vi "test_ServiceLocationPool_GetInvalidServiceTwice_DoesNotCacheInvalidData.vi"(8 "error in (no error)":errorcluster) -> (0 "error out":errorcluster, 2 "result":string, 3 "pass":bool)   [LabVIEW 2020, in "MeasurementServerTests.lvlib"]
uses:
  MeasurementServerTests.lvlib
  Runtime/MeasurementLink Discovery/MeasurementLink Discovery.lvlib
  Runtime/MeasurementLink Discovery Client/RPC Messages/ni_measurementlink_discovery_v1_ResolveServiceRequest.ctl
  Runtime/MeasurementLink Discovery Client/MeasurementLink Discovery Client.lvlib
  Runtime/MeasurementLink Discovery/Service Location FGV Action.ctl
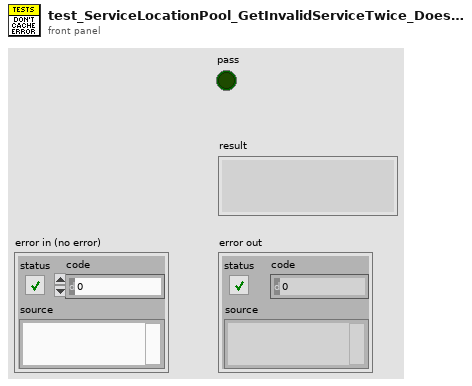
[diagram p1: front panel]
types:
  T1 = typedef "MeasurementLink Discovery Client.lvlib/ni_measurementlink_discovery_v1_ResolveServiceRequest.ctl" = cluster{"provided_interface":string, "service_class":string}
  T2 = typedef "MeasurementLink Discovery.lvlib/Service Location FGV Action.ctl" = enum16{"Get Service Location", "Reresolve Service Location"}
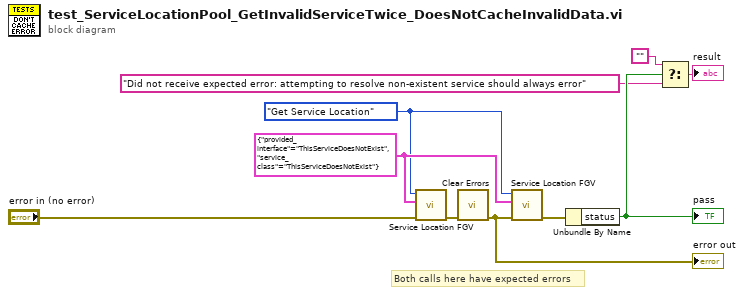
[diagram p0: block diagram]
diagram:
  w9 = T1 {"provided_interface"="ThisServiceDoesNotExist", "service_class"="ThisServiceDoesNotExist"} ("Resolve Service Request")
  w8 = Service_Location_FGV_Action."Get Service Location" ("Action")
  # "Both calls here have expected errors"
  n1 = call "Service Location FGV.vi"("error in"="error in (no error)", "resolve service request"=w9, "action"=w8) -> ("error out"=w6:errorcluster)  [unwired: 6 in, 2 out]
  n2 = call <vilib>:"Clear Errors.vi"("error in (no error)"=w6) -> ("error out"=w1:errorcluster)  [unwired: 5 in, 1 out]
  "error out" <- w1
  n3 = call "Service Location FGV.vi"("error in"=w1, "resolve service request"=w9, "action"=w8) -> ("error out"=w5:errorcluster)  [unwired: 6 in, 2 out]
  n4 = Unbundle By Name(w5) -> ("status"=w4:bool)
  "pass" <- w4
  n5 = Select(t="", s=w4, f="Did not receive expected error: attempting to resolve non-existent service should always error") -> (s? t:f=→"result":string)
